vi "initialize.vi"(0 "HGF_DSCService.lvclass":refnum<class "HGF_DSCService.lvclass">, 3 "initializationData":variant, 5 "error in (no error)":errorcluster, 7 "binaryString":string, 8 "I8 Array":i8[](array[numeric]), 9 "prependSize? (T)":bool, 11 "byteOrder (0:big-endian, network order)":T1(ring)) -> (14 "HGF_DSCService.lvclass":refnum<class "HGF_DSCService.lvclass">, 17 "found?":bool, 19 "error out":errorcluster)   [LabVIEW 2012, in "HGF_DSC.lvlib" / "HGF_DSCService.lvclass"]
uses:
  HGF_DSCService.lvclass
  HGF_DSCService.lvclass/HGF_DSCService.ctl
  HGF_SV/HGF_SVService/HGF_SVService.lvclass
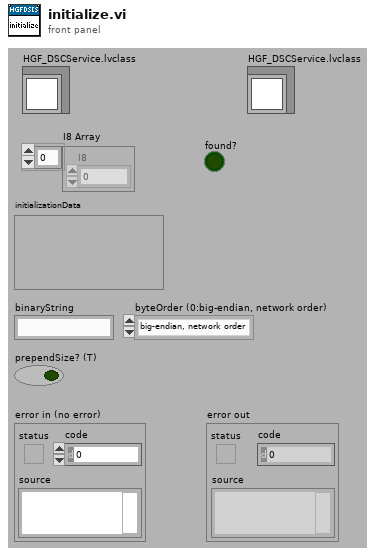
[diagram p1: front panel]
types:
  T1 = enum16{"big-endian, network order", "native, host order", "little-endian"}
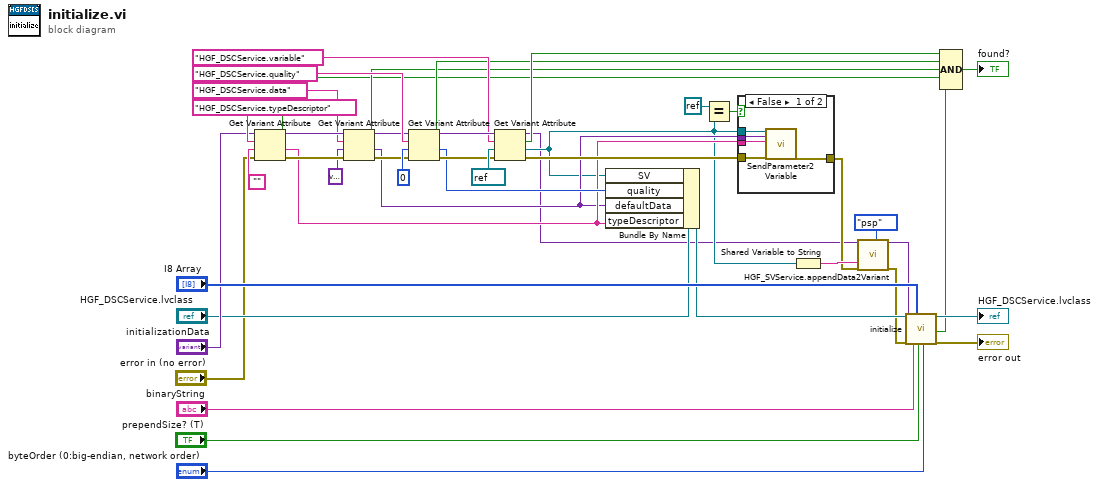
[diagram p0: block diagram]
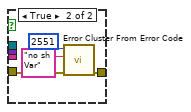
[diagram p2: hidden frame]
diagram:
  n1 = Get Variant Attribute(Variant="initializationData", name="HGF_DSCService.typeDescriptor", default value (empty Variant)="" ("typeDescriptor"), error in="error in (no error)") -> (duplicate Variant=w35:variant, found=w21:bool, value=w18:string, error out=w36:errorcluster)
  n2 = Get Variant Attribute(Variant=w35, name="HGF_DSCService.data", default value (empty Variant)=variant ("defaultData"), error in=w36) -> (duplicate Variant=w32:variant, found=w22:bool, value=w17:variant, error out=w31:errorcluster)
  n3 = Get Variant Attribute(Variant=w32, name="HGF_DSCService.quality", default value (empty Variant)=0 ("defaultQuality"), error in=w31) -> (duplicate Variant=w29:variant, found=w23:bool, value=w25:i32, error out=w28:errorcluster)
  n4 = Get Variant Attribute(Variant=w29, name="HGF_DSCService.variable", default value (empty Variant)=refnum<k21> refnum ("Shared Variable"), error in=w28) -> (duplicate Variant=w1:variant, found=w24:bool, value=w15:refnum<k21>, error out=w19:errorcluster)
  n5 = Bundle By Name(cluster="HGF_DSCService.lvclass", "SV"=w15, "quality"=w25, "defaultData"=w17, "typeDescriptor"=w18) -> (w7:refnum<class "HGF_DSCService.lvclass">)
  n6 = Equal?(x=refnum<k21> refnum, y=w15) -> (x = y?=w16:bool)
  n7 = case shown="False" w16 {
    tunnel: w19 -> [w48 w49]
    tunnel: [w47 w52] -> w5
    tunnel: w18 -> [w46 _]
    tunnel: w17 -> [w45 _]
    tunnel: w15 -> [w44 _]
    frame False {
      n8 = call "SendParameter2Variable.vi"("Shared Variable"=w44, "Parameter"=w45, "typeDescriptor"=w46, "error in (no error)"=w48) -> ("error out"=w47:errorcluster)  [unwired: 1 in, 14 out]
    }
    frame True {
      n9 = call <vilib>:"Error Cluster From Error Code.vi"("error in (no error)"=w49, "error message (\"\")"="no sh Var" ("error message (\"\")"), "error code (0)"=2551) -> ("error out"=w52:errorcluster)  [unwired: 1 in, 5 out]
    }
  }
  n10 = Shared Variable to String(1:w15) -> (0:w13:string)
  n11 = call "HGF_SVService.appendData2Variant.vi"("initData"=w1, "variable"=w13, "error in (no error)"=w5, "protocol"=enum8{"psp", "opc"}."psp") -> ("dup initData"=w11:variant, "error out"=w4:errorcluster)  [unwired: 3 in, 11 out]
  n12 = call-parent "initialize.vi"("HGF_SV.lvlib:HGF_SVService.lvclass"=w7, "initializationData"=w11, "error in (no error)"=w4, "binaryString"="binaryString", "I8 Array"="I8 Array", "prependSize? (T)"="prependSize? (T)", "byteOrder (0:big-endian, network order)"="byteOrder (0:big-endian, network order)") -> ("dup HGF_SV.lvlib:HGF_SVService.lvclass"=→"HGF_DSCService.lvclass":refnum<class "HGF_DSCService.lvclass">, "found?"=w6:bool, "error out"=→"error out":errorcluster)  [unwired: 10 out]
  n13 = Compound Arithmetic op=AND(w24, w23, w22, w21, w6) -> (→"found?":bool)
